vi "Parse Generic I2C Linux.vi"(10 "Bytes in":u8[](array[numeric]), 11 "pcap Parse and Build in":refnum<class "pcap_Parse_Build_CIF.lvclass">) -> (0 "Bus":u8 format="%.0x", 1 "7 bit Address":u8, 2 "Payload":u8[](array[numeric]) format="%.0x", 3 "pcap Parse and Build out":refnum<class "pcap_Parse_Build_CIF.lvclass">, 5 "Read":bool, 6 "TAI Time (ns)":i64)   [LabVIEW 2021, in "pcap_Parse_Build_CIF.lvclass"]
uses:
  pcap_Parse_Build_CIF.lvclass
  pcap_Parse_Build_CIF.lvclass/pcap_Parse_Build_CIF.ctl
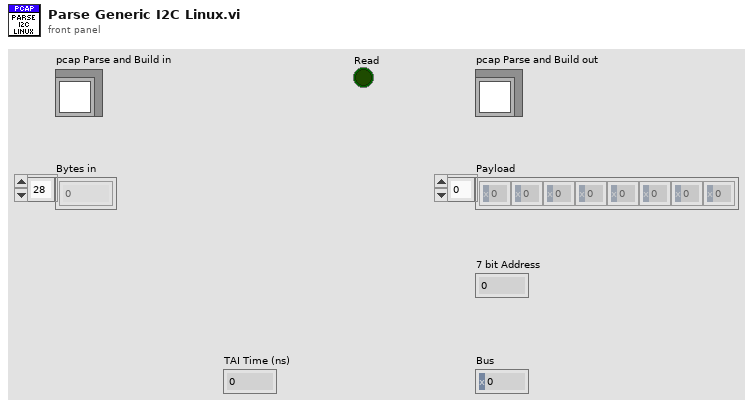
[diagram p1: front panel]
types:
  T1 = typedef "pcap_Parse_Build_CIF.lvclass/Packet Header.ctl" = cluster{"Timestamp (s)":u32, "Timestamp (ns)":u32, "Inc Length":u32, "Orig Length":u32}
  T2 = typedef "pcap_Parse_Build_CIF.lvclass/I2C Linux Header.ctl" = cluster{"Bus Number and Event Flag":u8, "Flags":u32, "HW Address":u8}
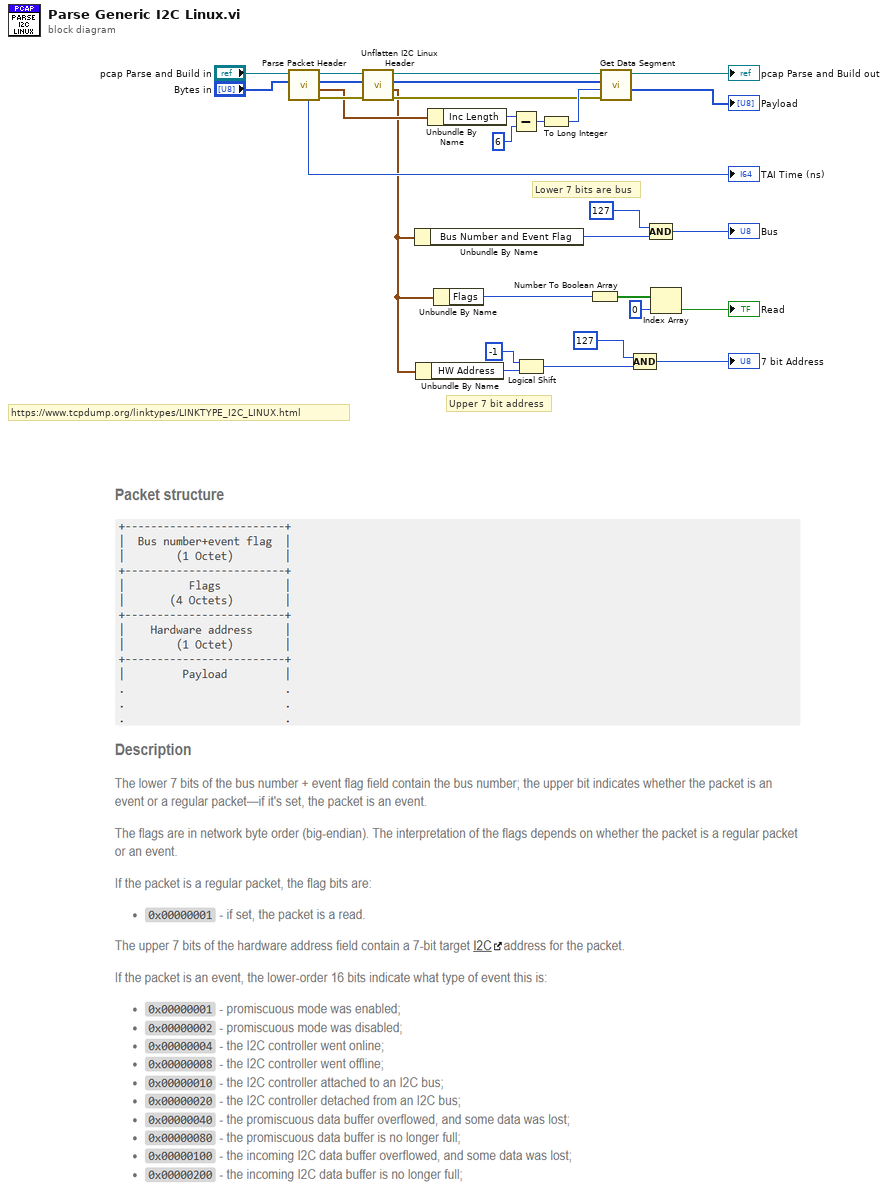
[diagram p0: block diagram]
diagram:
  # "Upper 7 bit address"
  # "https://www.tcpdump.org/linktypes/LINKTYPE_I2C_LINUX.html"
  # "Lower 7 bits are bus"
  n1 = call "Parse Packet Header.vi"("Bytes in"="Bytes in", "pcap Parse and Build in"="pcap Parse and Build in") -> ("error out"=w13:errorcluster, "Packet Header"=w11:T1, "Bytes out"=w17:u8[], "pcap Parse and Build out"=w16:refnum<class "pcap_Parse_Build_CIF.lvclass">, "TAI Time (ns)"=→"TAI Time (ns)":i64)  [unwired: 4 in, 1 out]
  n2 = call "Unflatten I2C Linux Header.vi"("error in (no error)"=w13, "Bytes in"=w17, "pcap Parse and Build in"=w16) -> ("error out"=w12:errorcluster, "I2C Lunix Header Out"=w6:T2, "Bytes out"=w14:u8[], "pcap Parse and Build out"=w15:refnum<class "pcap_Parse_Build_CIF.lvclass">)  [unwired: 5 in]
  n3 = Unbundle By Name(w6) -> ("Bus Number and Event Flag"=w7:u8)
  n4 = Unbundle By Name(w6) -> ("HW Address"=w4:u8)
  n5 = Unbundle By Name(w11) -> ("Inc Length"=w10:u32)
  n6 = Unbundle By Name(w6) -> ("Flags"=w27:u32)
  n7 = Subtract(x=w10, y=u32 6) -> (x-y=w9:u32)
  n8 = Logical Shift(y=i16 -1, x=w4) -> (x << y=w2:u8)
  n9 = To Long Integer(number=w9) -> (32bit integer=w23:i32)
  n10 = Number To Boolean Array(number=w27) -> (Boolean array=w26:bool[])
  n11 = call "Get Data Segment.vi"("error in (no error)"=w12, "Length"=w23, "Bytes in"=w14, "pcap Parse and Build in"=w15) -> ("Data Segment"=→"Payload":u8[], "pcap Parse and Build out"=→"pcap Parse and Build out":refnum<class "pcap_Parse_Build_CIF.lvclass">)  [unwired: 4 in, 2 out]
  n12 = Compound Arithmetic op=AND(u8 127 ("number"), w2) -> (→"7 bit Address":u8)
  n13 = Compound Arithmetic op=AND(u8 127 ("number"), w7) -> (→"Bus":u8)
  n14 = Index Array(array=w26, index=0) -> (element=→"Read":bool)
